vi "Flatten.vi"(8 "error in (no error)":errorcluster, 9 "Attributes":string[](array[string]), 10 "Pretty Print?":bool, 11 "JSON Scalar in":refnum<class "JSON Scalar.lvclass">) -> (0 "error out":errorcluster, 2 "String":string)   [LabVIEW 2011, in "JSON Scalar.lvclass"]
doc: "Converts an <b>JSON Scalar</b> into <b>String</b>. Use <b>Pretty Print?</b> to auto-indent and distribute the string over different lines.\n\nCopyright 2012 James David Powell, Shaun Rumbell and Ton Plomp\nMore information on http://lavag.org/topic/16217-cr-json-labview"
uses:
  JSON Scalar.lvclass
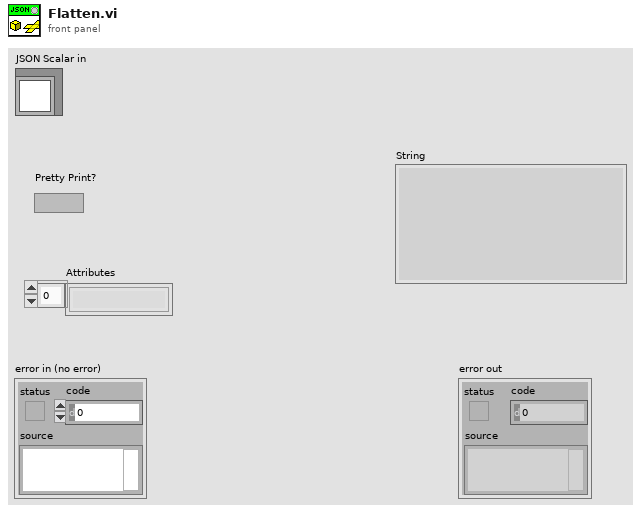
[diagram p1: front panel]
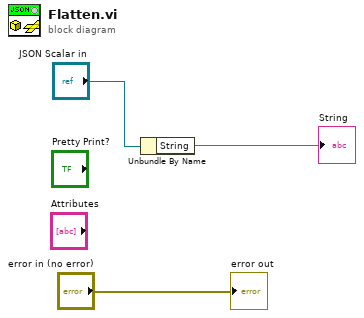
[diagram p0: block diagram]
diagram:
  n1 = Unbundle By Name("JSON Scalar in") -> ("String"=→"String":string)
  "error out" <- "error in (no error)"
